vi "Add Address.vi"(8 "error in (no error)":errorcluster, 11 "Node Ptr":u64 format="%.0x") -> (0 "error out":errorcluster)   [LabVIEW 2013, in "J1939 Addon System Explorer.lvlib"]
uses:
  J1939 Addon System Explorer.lvlib
  <vilib>/NI Veristand/Custom Device API/Custom Device Channel.ctl
  <vilib>/NI Veristand/Custom Device API/Custom Device Channel Type.ctl
  Shared/SubVIs/Constants.vi
  <vilib>/NI Veristand/Custom Device API/Set Item Property (Variant).vi
  Shared/J1939 Addon Shared.lvlib
  <vilib>/NI Veristand/Custom Device API/Custom Device API.lvlib
panel:
  in  "Tag":string
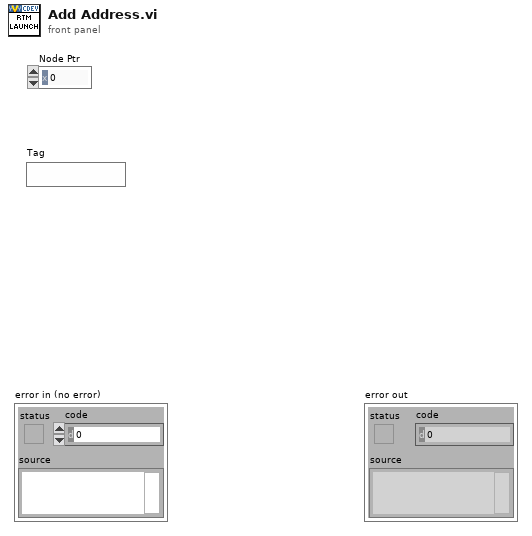
[diagram p1: front panel]
types:
  T1 = typedef "Custom Device API.lvlib/Custom Device Item Ref.ctl" = u64
  T2 = typedef "J1939 Addon Shared.lvlib/Monitor Settings.ctl" = cluster{"J1939 Network Address":u8, "Name":u64}
  T3 = typedef "Custom Device API.lvlib/Custom Device Channel.ctl" = cluster{"Type":T4, "Units":string, "Default Value":dbl, "Faultable":bool, "Scalable":bool}
  T4 = typedef "Custom Device API.lvlib/Custom Device Channel Type.ctl" = enum16{"Input", "Output"}
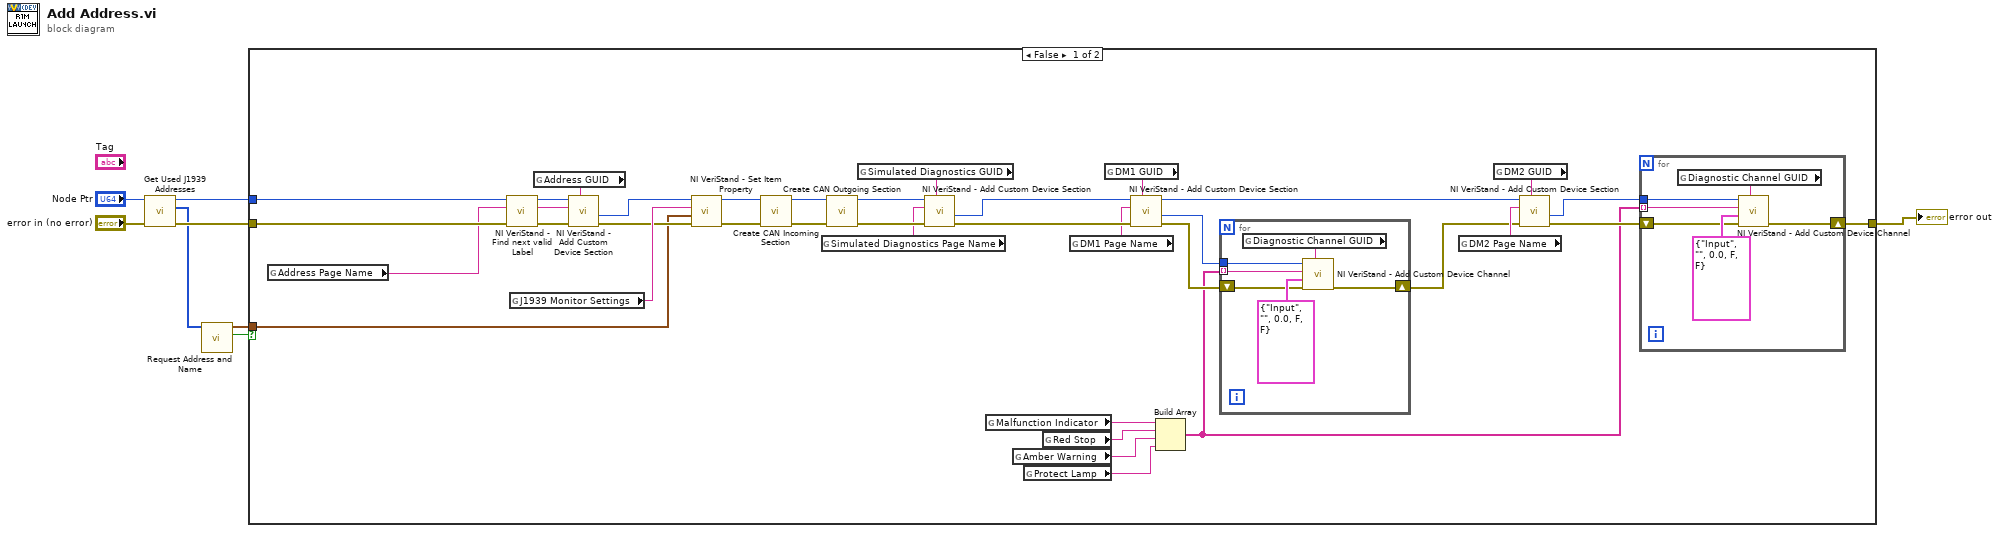
[diagram p0: block diagram]
diagram:
  n1 = call "Get Used J1939 Addresses.vi"("error in (no error)"="error in (no error)", "Node Ptr"="Node Ptr") -> ("error out"=w2:errorcluster, "Addresses"=w1:u8[], "Item Ref out"=w3:T1)  [unwired: 7 in]
  n2 = call "Request Address and Name.vi"("Used Addresses"=w1) -> ("Cancel out"=w7:bool, "J1939 Monitor Settings"=w6:T2)  [unwired: 9 in]
  n3 = case shown="False" w7 {
    tunnel: w3 -> [w42 _]
    tunnel: w2 -> [w10 w58]
    tunnel: [w18 w58] -> w8
    tunnel: w6 -> [w11 _]
    frame False {
      n4 = global read "Constants.vi" "Address Page Name"() -> (w9:string)
      n5 = call <vilib>:"NI VeriStand - Find next valid Label.vi"("error in (no error)"=w10, "Label"=w9, "Item Ref in"=w42) -> ("error out"=w40:errorcluster, "Label out"=w39:string, "Item Ref out"=w41:T1)  [unwired: 4 in, 2 out]
      n6 = global read "Constants.vi" "J1939 Monitor Settings"() -> (w16:string)
      n7 = global read "Constants.vi" "Address GUID"() -> (w43:string)
      n8 = call <vilib>:"NI VeriStand - Add Custom Device Section.vi"("GUID (Default Section)"=w43, "error in (no error)"=w40, "Section Name"=w39, "Parent Ref in"=w41) -> ("error out"=w15:errorcluster, "Section Ptr"=w13:T1)  [unwired: 4 in, 2 out]
      n9 = call-poly <vilib>:"NI VeriStand - Set Item Property.vi"("error in (no error)"=w15, "Value"=w11, "Property Name"=w16, "Item Ref in"=w13) -> ("error out"=w14:errorcluster, "Item Ref out"=w12:T1)  [unwired: 5 in, 1 out]
      n10 = call "Create CAN Incoming Section.vi"("error in (no error)"=w14, "Device Item Ref in"=w12) -> ("error out"=w45:errorcluster, "Device Item Ref Out"=w44:T1)  [unwired: 8 in]
      n11 = global read "Constants.vi" "Simulated Diagnostics Page Name"() -> (w35:string)
      n12 = call "Create CAN Outgoing Section.vi"("error in (no error)"=w45, "Parent Ref in"=w44) -> ("error out"=w36:errorcluster, "Parent Ref out"=w37:T1)  [unwired: 8 in]
      n13 = global read "Constants.vi" "Simulated Diagnostics GUID"() -> (w38:string)
      n14 = call <vilib>:"NI VeriStand - Add Custom Device Section.vi"("GUID (Default Section)"=w38, "error in (no error)"=w36, "Section Name"=w35, "Parent Ref in"=w37) -> ("error out"=w34:errorcluster, "Section Ptr"=w33:T1)  [unwired: 4 in, 2 out]
      n15 = global read "Constants.vi" "Malfunction Indicator"() -> (w28:string)
      n16 = global read "Constants.vi" "Amber Warning"() -> (w26:string)
      n17 = global read "Constants.vi" "Protect Lamp"() -> (w25:string)
      n18 = global read "Constants.vi" "Red Stop"() -> (w27:string)
      n19 = global read "Constants.vi" "DM1 Page Name"() -> (w31:string)
      n20 = global read "Constants.vi" "DM1 GUID"() -> (w32:string)
      n21 = call <vilib>:"NI VeriStand - Add Custom Device Section.vi"("GUID (Default Section)"=w32, "error in (no error)"=w34, "Section Name"=w31, "Parent Ref in"=w33) -> ("error out"=w24:errorcluster, "Section Ptr"=w22:T1, "Parent Ref out"=w21:T1)  [unwired: 4 in, 1 out]
      n22 = Build Array(w28, w27, w26, w25) -> (w17:string[])
      n23 = for {
        tunnel: w22 -> [w53]
        shift-right: [w54] -> w23
        shift-left: w24 -> [w55]
        tunnel: w17 -> [w52] mode=indexing
        n24 = global read "Constants.vi" "Diagnostic Channel GUID"() -> (w57:string)
        n25 = call <vilib>:"NI VeriStand - Add Custom Device Channel.vi"("GUID (Default Channel)"=w57, "error in (no error)"=w55, "Channel"=T3 {"Type"=enum."Input", "Units"="", "Default Value"=0.0, "Faultable"=FALSE, "Scalable"=FALSE}, "Channel Name"=w52, "Parent Ref in"=w53) -> ("error out"=w54:errorcluster)  [unwired: 3 in, 3 out]
      }
      n26 = global read "Constants.vi" "DM2 Page Name"() -> (w30:string)
      n27 = global read "Constants.vi" "DM2 GUID"() -> (w29:string)
      n28 = call <vilib>:"NI VeriStand - Add Custom Device Section.vi"("GUID (Default Section)"=w29, "error in (no error)"=w23, "Section Name"=w30, "Parent Ref in"=w21) -> ("error out"=w19:errorcluster, "Section Ptr"=w20:T1)  [unwired: 4 in, 2 out]
      n29 = for {
        tunnel: w20 -> [w47]
        shift-right: [w48] -> w18
        shift-left: w19 -> [w49]
        tunnel: w17 -> [w46] mode=indexing
        n30 = global read "Constants.vi" "Diagnostic Channel GUID"() -> (w51:string)
        n31 = call <vilib>:"NI VeriStand - Add Custom Device Channel.vi"("GUID (Default Channel)"=w51, "error in (no error)"=w49, "Channel"=T3 {"Type"=enum."Input", "Units"="", "Default Value"=0.0, "Faultable"=FALSE, "Scalable"=FALSE}, "Channel Name"=w46, "Parent Ref in"=w47) -> ("error out"=w48:errorcluster)  [unwired: 3 in, 3 out]
      }
    }
    frame True {
    }
  }
  "error out" <- w8
